vi "Get Elapsed Time (SubVI).vi"(8 "Go":bool, 11 "Experiment Time (S)":dbl) -> (0 "Done":bool, 3 "Time Status":string="Camera Connected")   [LabVIEW 2020]
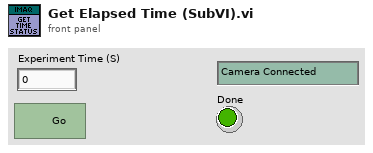
[diagram p1: front panel]
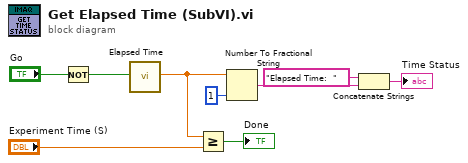
[diagram p0: block diagram]
diagram:
  n1 = Not(x="Go") -> (.not. x?=w1:bool)
  n2 = call "Elapsed Time"("Reset"=w1) -> ("Elapsed Time (s)"=w5:dbl)  [unwired: 11 in, 7 out]
  n3 = Greater Or Equal?(x=w5, y="Experiment Time (S)") -> (x >= y?=→"Done":bool)
  n4 = Number To Fractional String(number=w5, precision (6)=i16 1) -> (F-format string=w6:string)  [unwired: 2 in]
  n5 = Concatenate Strings("Elapsed Time:  " ("string"), w6) -> (→"Time Status":string)
